vi "MDAQ_GetCalibrationArray.vi"(6 "Fit Select":bool, 8 "Mirror Fit":T2, 9 "Fit":T2, 10 "Cluster In":T1 {"GATESTOP" format="%04x"; "GATESTRT" format="%04x"; "AMPLITUDE" format="%04x"; "M_CYCLES" format="%04x"; "N_CYCLES" format="%04x"; "STEP" format="%04x"; "BASE" format="%04x"; "CHAN" format="%04x"}) -> (2 "Cluster Out":T1 {"GATESTOP" format="%04x"; "GATESTRT" format="%04x"; "AMPLITUDE" format="%04x"; "M_CYCLES" format="%04x"; "N_CYCLES" format="%04x"; "STEP" format="%04x"; "BASE" format="%04x"; "CHAN" format="%04x"})   [LabVIEW 2021]
uses:
  Status_Cluster.ctl
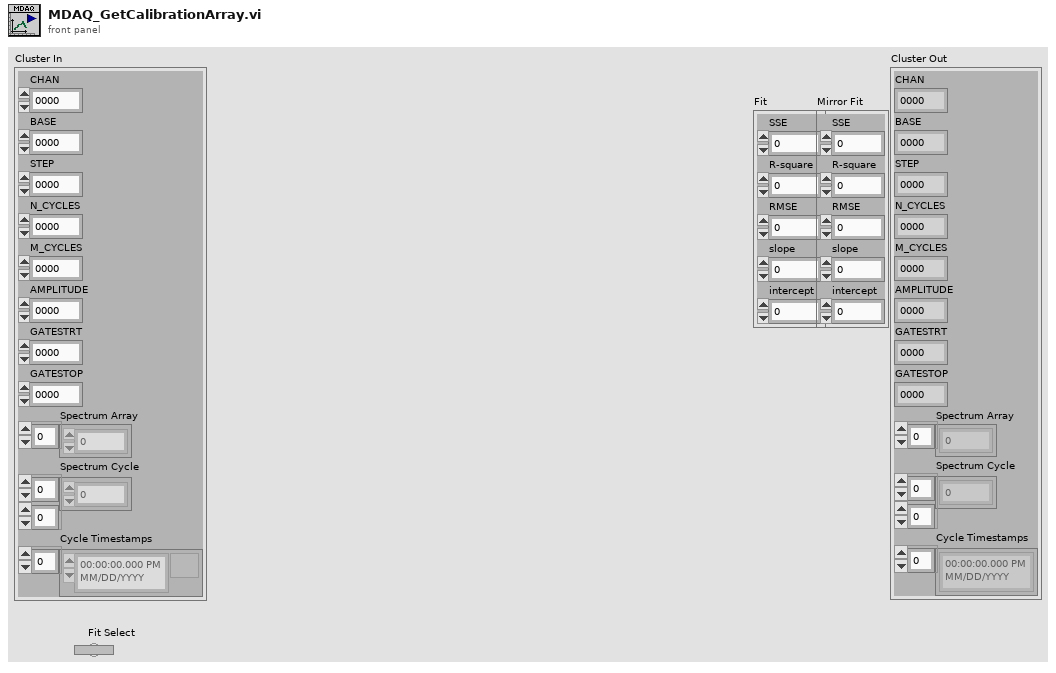
[diagram p1: front panel]
types:
  T1 = typedef "Status_Cluster.ctl" = cluster{"CHAN":u32, "BASE":u32, "STEP":u32, "N_CYCLES":u32, "M_CYCLES":u32, "AMPLITUDE":u32, "GATESTRT":u32, "GATESTOP":u32, "Spectrum Array":u32[], "Spectrum Cycle":u32[][], "Cycle Timestamps":timestamp[]}
  T2 = cluster{"SSE":dbl, "R-square":dbl, "RMSE":dbl, "slope":dbl, "intercept":dbl}
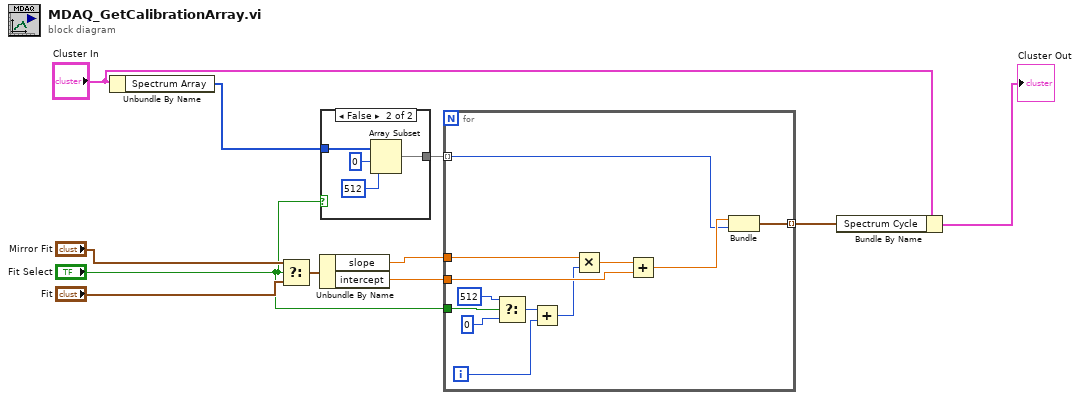
[diagram p0: block diagram]
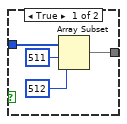
[diagram p2: hidden frame]
diagram:
  n1 = Unbundle By Name("Cluster In") -> ("Spectrum Array"=w3:u32[])
  n2 = Select(t="Mirror Fit", s="Fit Select", f="Fit") -> (s? t:f=w9:T2)
  n3 = Unbundle By Name(w9) -> ("slope"=w8:dbl, "intercept"=w7:dbl)
  n4 = case shown="False" "Fit Select" {
    tunnel: w3 -> [w15 w19]
    tunnel: [w14 w18] -> w2
    frame True {
      n5 = Array Subset(array=w15, index=511, length=512) -> (w14:u32[])
    }
    frame False {
      n6 = Array Subset(array=w19, index=0, length=512) -> (w18:u32[])
    }
  }
  n7 = for {
    tunnel: w2 -> [w26] mode=indexing
    tunnel: w8 -> [w30]
    tunnel: w7 -> [w28]
    tunnel: [w31] -> w5 mode=indexing
    tunnel: "Fit Select" -> [w25]
    i -> [w21]
    n8 = Select(t=512, s=w25, f=0) -> (s? t:f=w23:i32)
    n9 = Add(x=w23, y=w21) -> (x+y=w20:i32)
    n10 = Multiply(x=w30, y=w20) -> (x*y=w29:dbl)
    n11 = Add(x=w29, y=w28) -> (x+y=w27:dbl)
    n12 = Bundle(w27, w26) -> (w31:cluster{dbl, u32})  [unwired: 1 in]
  }
  n13 = Bundle By Name(cluster="Cluster In", "Spectrum Cycle"=w5) -> (→"Cluster Out":T1)
